vi "LAB3_EXP02.vi"() -> ()   [LabVIEW 2015]
uses:
  <vilib>/measure/maspectr.llb/FFT Spectrum (Mag-Phase) for N Chan.vi
  <vilib>/measure/NI_MABase.lvlib
  <vilib>/measure/NI_MAPro.lvlib
panel:
  out "ml-mr final Graph":dynamicdata(graph)=[{"t0"=timestamp(0 s since 1904-01-01), "dt"=8.333333333333334e-06, "Y"=array[250 elements], "attributes"=variant("NI_ChannelName"=variant(string "Filtered (Filtered)"), "NI_OriginalChannelName"=variant(string "Filtered"))}]
  out "ml-mr initial Graph":dynamicdata(graph)=[{"t0"=timestamp(0 s since 1904-01-01), "dt"=8.333333333333334e-06, "Y"=array[250 elements], "attributes"=variant("NI_ChannelName"=variant(string "Filtered"))}]
  out "m2 FILTERED Graph":dynamicdata(graph)=[{"t0"=timestamp(0 s since 1904-01-01), "dt"=8.333333333333334e-06, "Y"=array[250 elements], "attributes"=variant("NI_ChannelName"=variant(string "Filtered"))}]
  out "2M2 FINAL  Graph":dynamicdata(graph)=[{"t0"=timestamp(0 s since 1904-01-01), "dt"=8.333333333333334e-06, "Y"=array[250 elements], "attributes"=variant("NI_ChannelName"=variant(string "Filtered (Filtered)"), "NI_OriginalChannelName"=variant(string "Filtered"))}]
  out "2M1 FINAL Graph":dynamicdata(graph)=[{"t0"=timestamp(0 s since 1904-01-01), "dt"=8.333333333333334e-06, "Y"=array[250 elements], "attributes"=variant("NI_ChannelName"=variant(string "Filtered (Filtered)"), "NI_OriginalChannelName"=variant(string "Filtered"))}]
  out "TRANSMITTED SIGNAL FINAL":cluster{"f0":dbl, "df":dbl, "magnitude":dbl[]}[](graph)=[{"f0"=0.0, "df"=480.0, "magnitude"=[0.0007812302888471505, 0.005192735308412077, 0.022964038836516484, 0.055172832850028455, 0.0962082338664353, 0.12781146869157195, 0.11196728052098676, 0.10391745118762145, 0.10163007377423373, 0.05314927127751649, 0.05126786280355977, 0.14213910446934636, 0.1474122605939654, 0.08031550706894412, 0.05037166667441142, 0.07749498628191945, 0.053557130364944826, 0.015198074947686588, 0.05502979779845201, 0.1511423251629442, 0.2054879311904084, 0.20155154324885266, 0.15570575808605233, 0.0722207057749931, 0.07245773558188938, 0.08769047777546983, 0.059342810192852334, 0.031127048020854794, 0.04267785548732679, 0.04000063794439573, 0.022699422379406507, 0.007959116036291857, 0.0014345821084623337, 0.00024114546384851305, 0.00025884030262100354, 0.0002848742419576737, 0.0005312197191175263, 0.0014937138944982576, 0.00911926879825831, 0.056487940403503994, 0.06314514253679557, 0.015236393021688522, 0.0018549053182662038, 0.0005936776599360025, 0.0002689671634657977, 0.00017521725852346742, 0.0002559420226017131, 0.0007007312772380565, 0.0018335145031912032, 0.003779295397525955, 0.0060748980486918635, 0.0076665558479664195, 0.006810990033234126, 0.002923814166400638, 0.009921911819060223, 0.016775837079741788, 0.014485917847960484, 0.0047439495154453105, 0.005377245062734432, 0.012260691920751032, 0.017947773762337124, 0.017469670513619452, 0.009310637509257208, 0.021673893823090467, 0.025441480983432605, 0.0017711740355476652, 0.027580141788499858, 0.03177004336830579, 0.01031716388906587, 0.023514528583362847, 0.04237619048685987, 0.03402485209815197, 0.02376956951565321, 0.022688718342111336, 0.010704995101537058, 0.0052978319425557065, 0.007708495400157739, 0.00721195410372173, 0.003047266426781619, 0.0003282236041602661, 0.001866569132218354, 0.005932240728606129, 0.00819794083365282, 0.005821343418526996, 0.00744784505774242, 0.019274890167737573, 0.024436710080594087, 0.02834358710657392, 0.04249203272213193, 0.032230619620166184, 0.006058359366388453, 0.026494018043966484, 0.03258149257592319, 0.009219092504890265, 0.020240772720135775, 0.025733230282702548, 0.011122272497757109, 0.014926698318172884, 0.018851883597281124, 0.014385218258857805, 0.007838765087476825, 0.0016152496661014741, 0.01169852856275451, 0.017168579324866092, 0.012892255743778974, 0.003993487837137806, 0.005622557445093134, 0.0077658410339264345, 0.006768014795427597, 0.004554683939636923, 0.0023749303281198264, 0.0009445178837378146, 0.0003106089837972868, 0.00011434132495003295, 5.344034987124318e-05, 2.8513212948968436e-05, 1.688856862439638e-05, 1.077469594172098e-05, 7.242599002521258e-06, 5.052862149994133e-06, 3.616204374439302e-06, 2.629418911262323e-06, 1.929500585685826e-06, 1.4328539403396243e-06, 1.1145491075295667e-06]}]
  out "m1 FILTERED  Graph":dynamicdata(graph)=[{"t0"=timestamp(0 s since 1904-01-01), "dt"=8.333333333333334e-06, "Y"=array[250 elements], "attributes"=variant("NI_ChannelName"=variant(string "Filtered"))}]
  in  "K":dbl=0.1
  in  "phase":dbl=90.0 format="%.2p"
  in  "amplitude":dbl=1.0 format="%0.2p"
  in  "frequency":dbl=19000.0 format="%0.2p"
  in  "sampling info":cluster{"Fs":dbl, "#s":dbl}={"Fs"=120000.0, "#s"=250.0} {"Fs" format="%.2p"}
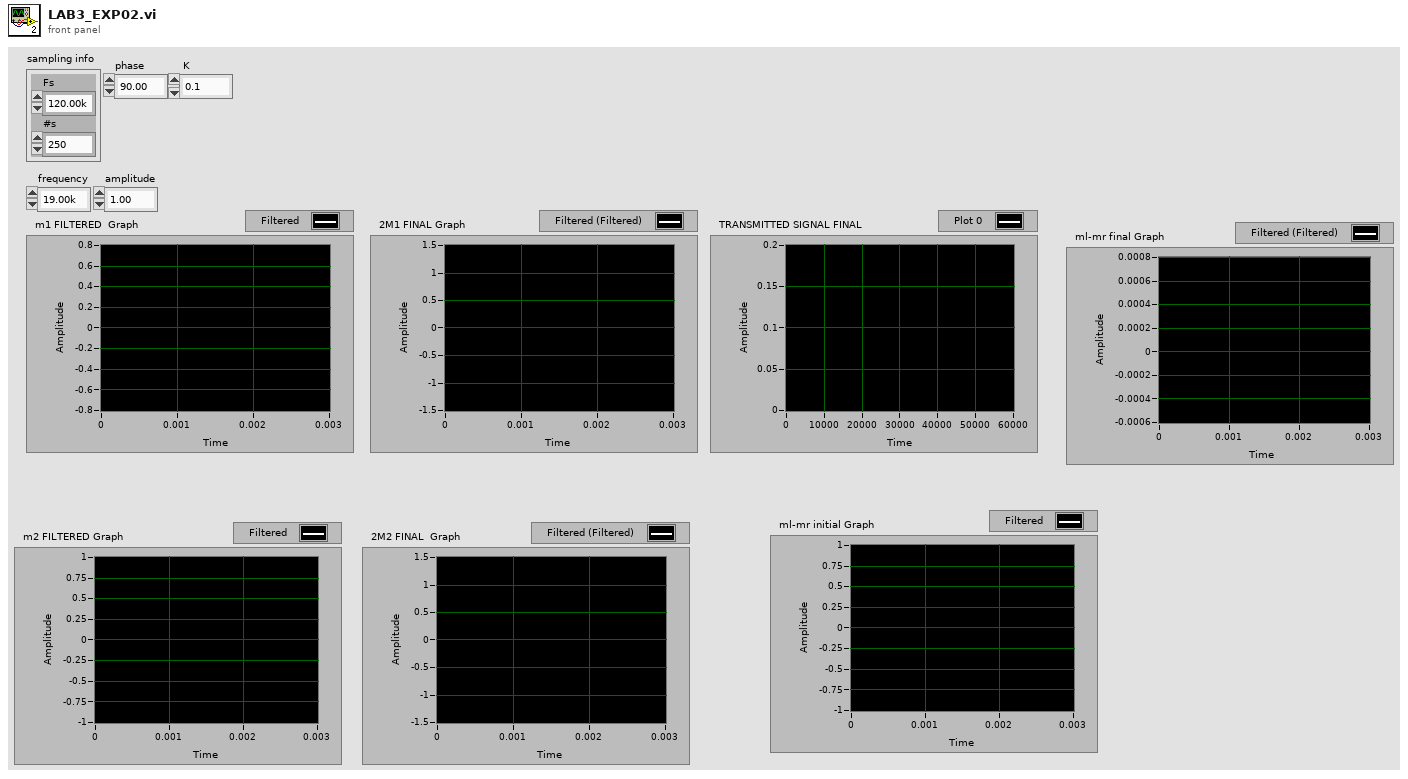
[diagram p1: front panel]
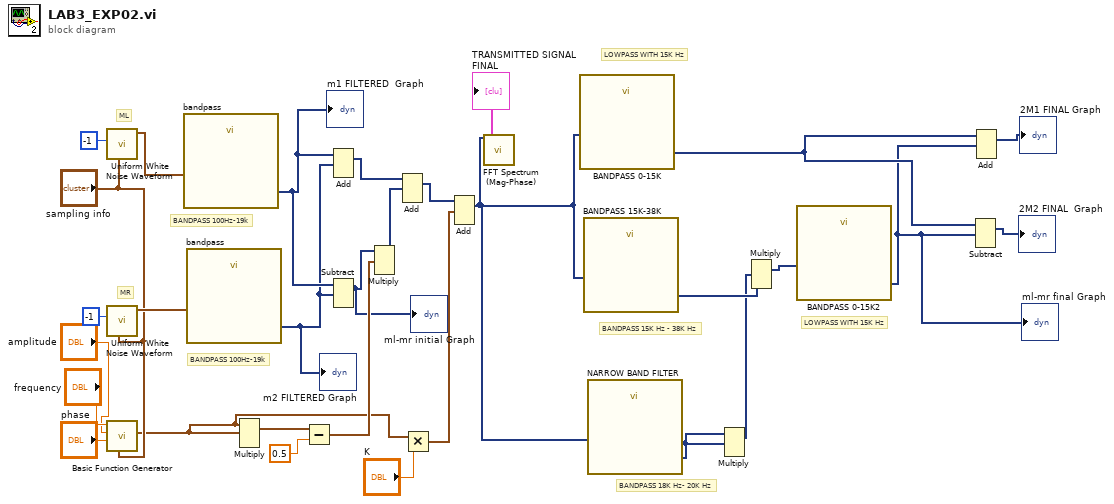
[diagram p0: block diagram]
diagram:
  # "LOWPASS WITH 15K Hz"
  # "BANDPASS 18K Hz- 20K Hz"
  # "BANDPASS 15K Hz - 38K Hz"
  # "LOWPASS WITH 15K Hz"
  # "MR"
  # "ML"
  # "BANDPASS 100Hz-19k"
  # "BANDPASS 100Hz-19k"
  n1 = call <vilib>:"Uniform White Noise Waveform.vi"("sampling info"="sampling info", "seed"=-1) -> ("signal out"=w29:waveform(dbl))  [unwired: 8 in, 1 out]
  n2 = call <vilib>:"Uniform White Noise Waveform.vi"("sampling info"="sampling info", "seed"=-1) -> ("signal out"=w30:waveform(dbl))  [unwired: 8 in, 1 out]
  n3 = call <vilib>:"Basic Function Generator.vi"("sampling info"="sampling info", "phase"="phase", "amplitude"="amplitude", "frequency"="frequency") -> ("signal out"=w14:waveform(dbl))  [unwired: 5 in, 2 out]
  n4 = call "bandpass"("Signal"=w29) -> ("Filtered Signal"=w15:dynamicdata)  [unwired: 9 in, 1 out]
  "m1 FILTERED  Graph" <- w15
  n5 = call "bandpass"("Signal"=w30) -> ("Filtered Signal"=w4:dynamicdata)  [unwired: 9 in, 1 out]
  "m2 FILTERED Graph" <- w4
  n6 = Multiply(1:w14, 2:w14) -> (0:w24:waveform(dbl))  [unwired: 1 in, 1 out]
  n7 = Subtract(x=w24, y=0.5) -> (x-y=w20:waveform(dbl))
  n8 = Add(1:w4, 2:w15) -> (0:w22:dynamicdata)  [unwired: 1 in, 1 out]
  n9 = Subtract(1:w4, 2:w15) -> (0:w2:dynamicdata)  [unwired: 1 in, 1 out]
  "ml-mr initial Graph" <- w2
  n10 = Multiply(1:w20, 2:w2) -> (0:w21:dynamicdata)  [unwired: 1 in, 1 out]
  n11 = Add(1:w21, 2:w22) -> (0:w17:dynamicdata)  [unwired: 1 in, 1 out]
  n12 = Multiply(x=w14, y="K") -> (x*y=w18:waveform(dbl))
  n13 = Add(1:w18, 2:w17) -> (0:w11:dynamicdata)  [unwired: 1 in, 1 out]
  n14 = call-poly <vilib>:"FFT Spectrum (Mag-Phase).vi"("time signals"=w11) -> ("magnitudes"=→"TRANSMITTED SIGNAL FINAL":cluster{"f0":dbl, "df":dbl, "magnitude":dbl[]}[])  [unwired: 6 in, 4 out]
  n15 = call "BANDPASS 0-15K"("Signal"=w11) -> ("Filtered Signal"=w6:dynamicdata)  [unwired: 9 in, 1 out]
  n16 = call "BANDPASS 15K-38K"("Signal"=w11) -> ("Filtered Signal"=w9:dynamicdata)  [unwired: 9 in, 1 out]
  n17 = call "NARROW BAND FILTER"("Signal"=w11) -> ("Filtered Signal"=w10:dynamicdata)  [unwired: 9 in, 1 out]
  n18 = Multiply(1:w10, 2:w10) -> (0:w8:dynamicdata)  [unwired: 1 in, 1 out]
  n19 = Multiply(1:w8, 2:w9) -> (0:w7:dynamicdata)  [unwired: 1 in, 1 out]
  n20 = call "BANDPASS 0-15K2"("Signal"=w7) -> ("Filtered Signal"=w1:dynamicdata)  [unwired: 9 in, 1 out]
  "ml-mr final Graph" <- w1
  n21 = Subtract(1:w1, 2:w6) -> (0:→"2M2 FINAL  Graph":dynamicdata)  [unwired: 1 in, 1 out]
  n22 = Add(1:w1, 2:w6) -> (0:→"2M1 FINAL Graph":dynamicdata)  [unwired: 1 in, 1 out]
